vi "TP STRING.vi"(10 "tpdata":string[](array[string])) -> (2 "TP OUT":string)   [LabVIEW 2018]
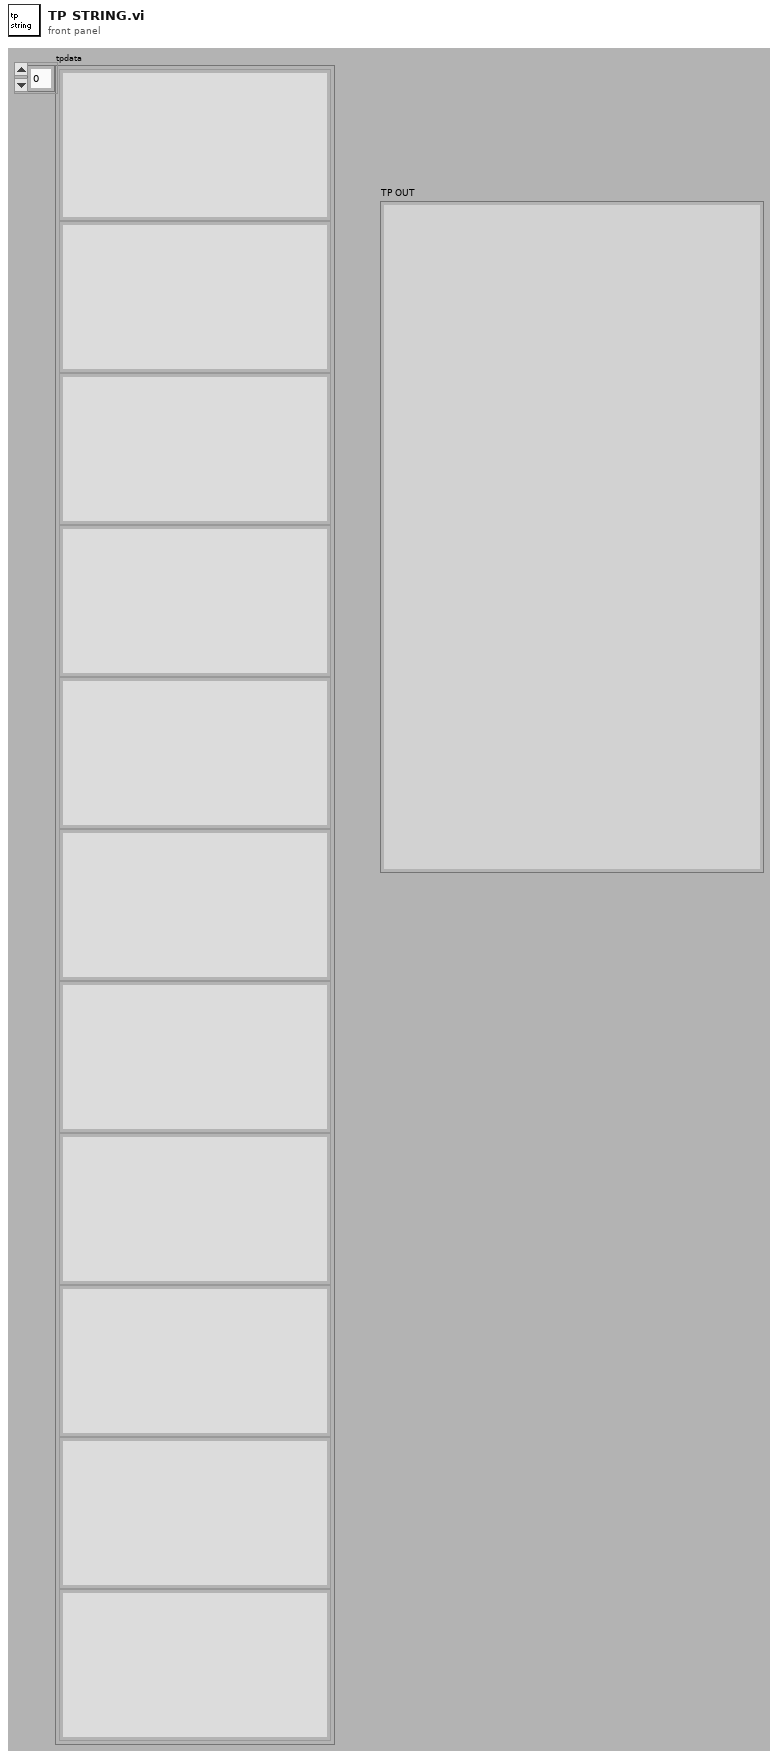
[diagram p1: front panel]
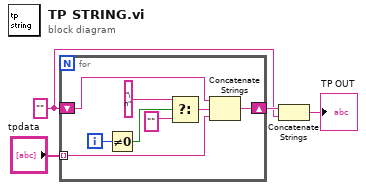
[diagram p0: block diagram]
diagram:
  w2 = "" ("genneral TP info")
  n1 = for {
    shift-right: [w11] -> w4
    shift-left: w2 -> [w12]
    tunnel: "tpdata" -> [w5] mode=indexing
    i -> [w10]
    n2 = Not Equal To 0?(x=w10) -> (x != 0?=w9:bool)
    n3 = Select(t="\n", s=w9, f="") -> (s? t:f=w6:string)
    n4 = Concatenate Strings(w12, w6, w5) -> (w11:string)
  }
  n5 = Concatenate Strings(w4, w2) -> (→"TP OUT":string)
